vi "Close.vi"(11 "Custom Device in":refnum<class "Template.lvclass">) -> (0 "error out":errorcluster, 3 "Custom Device out":refnum<class "Template.lvclass">)   [LabVIEW 2026, in "Template.lvlib" / "Template.lvclass"]
uses:
  Template.lvclass
  Template.lvclass/Template.ctl
  <userlib>/NIVS Inline Async API (Express)/_VS Inline Async API (Express)/VS Inline Async API (Express)/VS Inline Async API (Express).lvclass
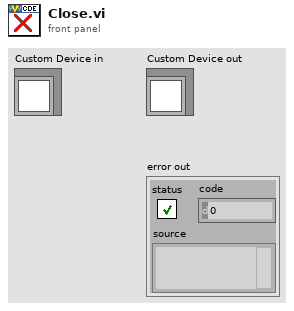
[diagram p1: front panel]
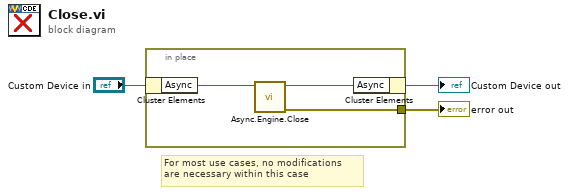
[diagram p0: block diagram]
diagram:
  # "For most use cases, no modifications \nare necessary within this case"
  n1 = in-place {
    in-place-border: [w6] -> w1
    n2 = in-place-cluster #1("Custom Device in") -> ("Async"=w5:refnum<class "VS Inline Async API (Express).lvclass">)
    n3 = call <userlib>:"Async.Engine.Close.vi"("Async in"=w5) -> ("error out"=w6:errorcluster, "Async out"=w4:refnum<class "VS Inline Async API (Express).lvclass">)  [unwired: 9 in]
    n4 = in-place-cluster #1("Async"=w4) -> (→"Custom Device out":refnum<class "Template.lvclass">)
  }
  "error out" <- w1
